vi "niDTS BT LE Tx Test Get Default Limits.vi"(0 "Dummy Test Handle In":T1, 11 "error in (no error)":errorcluster) -> (4 "Dummy Test Handle Out":T1, 6 "USL":T2, 8 "LSL":T2, 15 "error out":errorcluster)   [LabVIEW 2014, in "niDTS BT.lvlib"]
uses:
  niDTS BT.lvlib
  Includes/niDTS BT LE Tx Test INC Results.ctl
  Tx Test/Includes/niDTS BT Tx Test INC IBE Results.ctl
  Tx Test/Includes/niDTS BT Tx Test INC Character Results.ctl
  Tx Test/Includes/niDTS BT Tx Test INC CFO Resutls.ctl
  Tx Test/Includes/niDTS BT Tx Test INC TXP Results.ctl
  Tx Test/Includes/niDTS BT Tx Test INC Handle.ctl
  Tx Test/Objects/BASE_class/niDTS BT Tx Test.lvclass
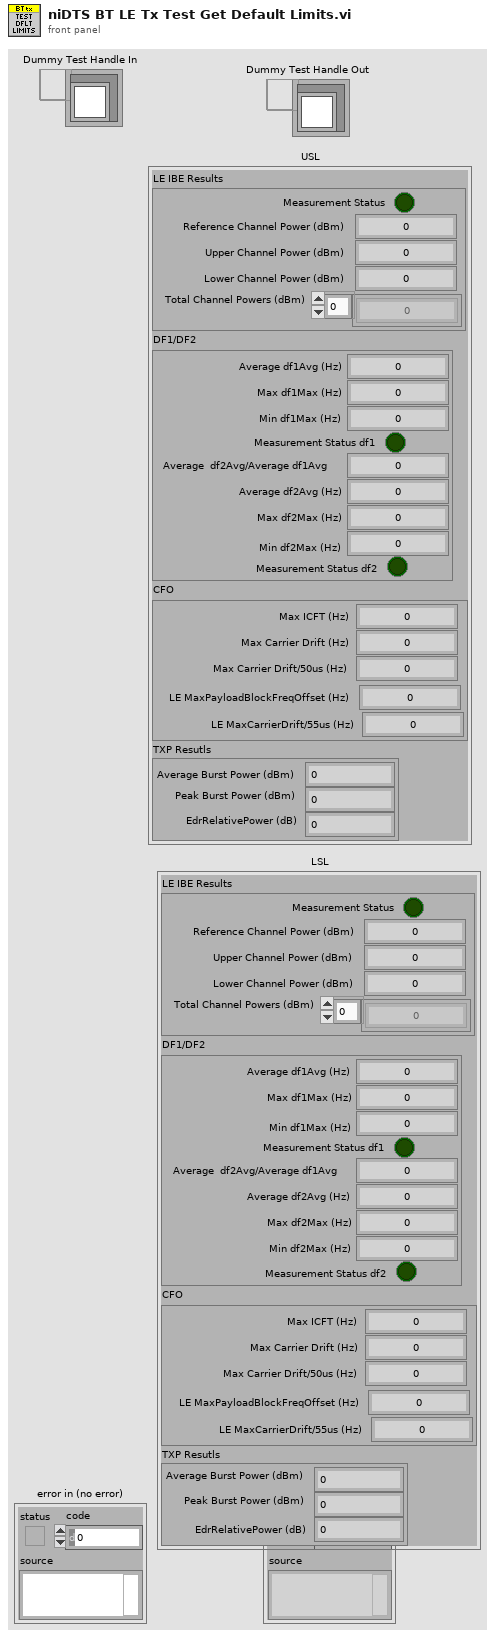
[diagram p1: front panel]
types:
  T1 = typedef "niDTS BT.lvlib/niDTS BT Tx Test INC Handle.ctl" = refnum<data-value>
  T2 = typedef "niDTS BT.lvlib/niDTS BT LE Tx Test INC Results.ctl" = cluster{"LE IBE Results":T3, "DF1/DF2":T4, "CFO":T5, "TXP Resutls":T6}
  T3 = typedef "niDTS BT.lvlib/niDTS BT Tx Test INC IBE Results.ctl" = cluster{"Measurement Status":bool, "Reference Channel Power (dBm)":dbl, "Upper Channel Power (dBm)":dbl, "Lower Channel Power (dBm)":dbl, "Total Channel Powers (dBm)":dbl[]}
  T4 = typedef "niDTS BT.lvlib/niDTS BT Tx Test INC Character Results.ctl" = cluster{"Average df1Avg (Hz)":dbl, "Max df1Max (Hz)":dbl, "Min df1Max (Hz)":dbl, "Measurement Status df1":bool, "Average  df2Avg/Average df1Avg":dbl, "Average df2Avg (Hz)":dbl, "Max df2Max (Hz)":dbl, "Min df2Max (Hz)":dbl, "Measurement Status df2":bool}
  T5 = typedef "niDTS BT.lvlib/niDTS BT Tx Test INC CFO Resutls.ctl" = cluster{"Max ICFT (Hz)":dbl, "Max Carrier Drift (Hz)":dbl, "Max Carrier Drift/50us (Hz)":dbl, "LE MaxPayloadBlockFreqOffset (Hz)":dbl, "LE MaxCarrierDrift/55us (Hz)":dbl}
  T6 = typedef "niDTS BT.lvlib/niDTS BT Tx Test INC TXP Results.ctl" = cluster{"Average Burst Power (dBm)":dbl, "Peak Burst Power (dBm)":dbl, "EdrRelativePower (dB)":dbl}
  T7 = typedef "niDTS BT.lvlib/niDTS BT Tx Test INC Results.ctl" = cluster{"IBE Results":T3, "OBW Resutls":T8, "TXP Resutls":T6, "DEVM":T9, "CF Stability":T10, "CFO":T5, "DF1/DF2":T4}
  T8 = typedef "niDTS BT.lvlib/niDTS BT Tx Test INC OBW Results.ctl" = cluster{"OBW (Hz)":dbl, "Start Frequency (Hz)":dbl, "Stop Frequency (Hz)":dbl}
  T9 = typedef "niDTS BT.lvlib/niDTS BT Tx Test INC DEVM Results.ctl" = cluster{"Average RMS DEVM (%)":dbl, "Max Peak DEVM (%)":dbl, "99% DEVM (%)":dbl}
  T10 = typedef "niDTS BT.lvlib/niDTS BT Tx Test INC CF Stability Results.ctl" = cluster{"Average Inital Freq Error (Hz)":dbl, "Max Initial Freq Error (Hz)":dbl, "Average Block Abs Freq Error (Hz)":dbl, "Max Block Abs Freq Error (Hz)":dbl, "Average Block Rel Freq Error (Hz)":dbl, "MaxBlockRel Freq Error (Hz)":dbl}
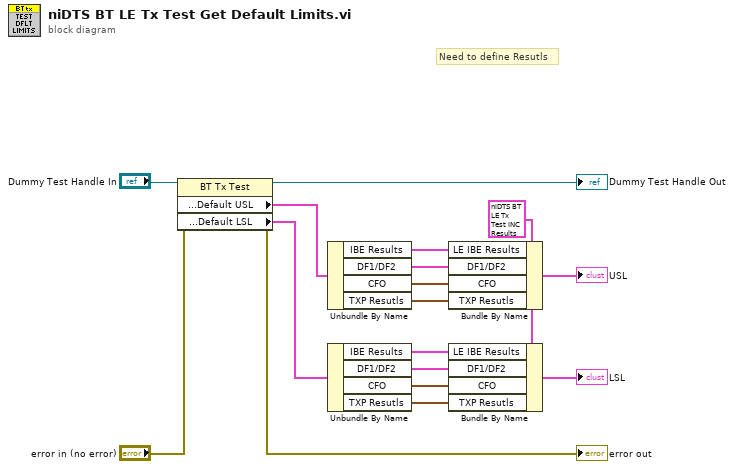
[diagram p0: block diagram]
diagram:
  w1 = T2 {"LE IBE Results"={"Measurement Status"=FALSE, "Reference Channel Power (dBm)"=0.0, "Upper Channel Power (dBm)"=0.0, "Lower Channel Power (dBm)"=0.0, "Total Channel Powers (dBm)"=[]}, "DF1/DF2"={"Average df1Avg (Hz)"=0.0, "Max df1Max (Hz)"=0.0, "Min df1Max (Hz)"=0.0, "Measurement Status df1"=FALSE, "Average  df2Avg/Average df1Avg"=0.0, "Average df2Avg (Hz)"=0.0, "Max df2Max (Hz)"=0.0, "Min df2Max (Hz)"=0.0, "Measurement Status df2"=FALSE}, "CFO"={"Max ICFT (Hz)"=0.0, "Max Carrier Drift (Hz)"=0.0, "Max Carrier Drift/50us (Hz)"=0.0, "LE MaxPayloadBlockFreqOffset (Hz)"=0.0, "LE MaxCarrierDrift/55us (Hz)"=0.0}, "TXP Resutls"={"Average Burst Power (dBm)"=0.0, "Peak Burst Power (dBm)"=0.0, "EdrRelativePower (dB)"=0.0}} ("USL")
  # "Need to define Resutls"
  n1 = property class="BT Tx Test"(reference="Dummy Test Handle In", error in="error in (no error)") -> (reference out=→"Dummy Test Handle Out":T1, error out=→"error out":errorcluster, "Properties:Default Limits:Default USL"=w15:T7, "Properties:Default Limits:Default LSL"=w3:T7)
  n2 = Unbundle By Name(w15) -> ("IBE Results"=w12:T3, "DF1/DF2"=w11:T4, "CFO"=w10:T5, "TXP Resutls"=w9:T6)
  n3 = Unbundle By Name(w3) -> ("IBE Results"=w5:T3, "DF1/DF2"=w6:T4, "CFO"=w7:T5, "TXP Resutls"=w8:T6)
  n4 = Bundle By Name(cluster=w1, "LE IBE Results"=w12, "DF1/DF2"=w11, "CFO"=w10, "TXP Resutls"=w9) -> (→"USL":T2)
  n5 = Bundle By Name(cluster=w1, "LE IBE Results"=w5, "DF1/DF2"=w6, "CFO"=w7, "TXP Resutls"=w8) -> (→"LSL":T2)
